vi "GUILib.find control by name.vi"(0 "control name":string, 1 "VIRef":refnum<vi>, 5 "error in (no error)":errorcluster) -> (14 "controlRef":refnum<vi>, 19 "error out":errorcluster)   [LabVIEW 2014, in "GUILib.lvlib"]
doc: "obtains the reference of a control of a VI"
uses:
  GUILib.lvlib
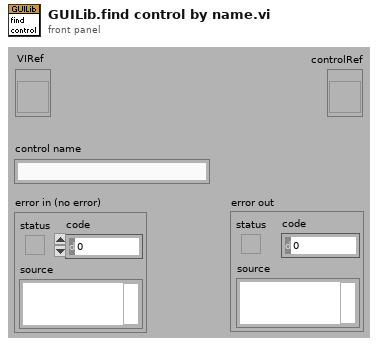
[diagram p1: front panel]
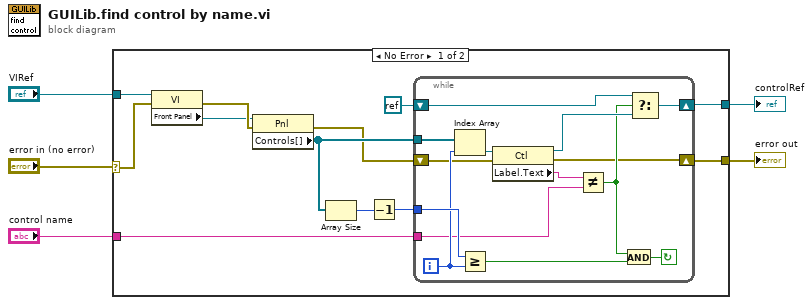
[diagram p0: block diagram]
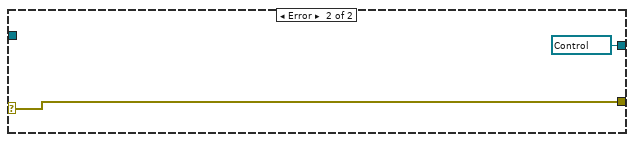
[diagram p2: hidden frame]
diagram:
  n1 = case shown="No Error" "error in (no error)" {
    selector: "error in (no error)" -> [w7 w33]
    tunnel: [w13 refnum<vi> refnum ("dup reference")] -> w5
    tunnel: [w10 w33] -> w4
    tunnel: "VIRef" -> [w9 _]
    tunnel: "control name" -> [w8 _]
    frame No Error {
      n2 = property on="Property Node" class="VI"(reference=w9, error in=w7) -> (error out=w17:errorcluster, "Front Panel"=w16:refnum<vi>)  [unwired: 1 out]
      n3 = property on="Property Node" class="Pnl"(reference=w16, error in=w17) -> (error out=w11:errorcluster, "Controls[]"=w14:refnum<vi>[])  [unwired: 1 out]
      n4 = Array Size(array=w14) -> (size(s)=w15:i32)
      n5 = Decrement(x=w15) -> (x-1=w12:i32)
      n6 = while {
        tunnel: w12 -> [w31]
        tunnel: w14 -> [w30]
        shift-right: [w26] -> w13
        shift-left: refnum<k0> refnum ("Not a Refnum Constant") -> [w25]
        shift-right: [w19] -> w10
        shift-left: w11 -> [w20]
        tunnel: w8 -> [w18]
        i -> [w29]
        stop <- w23 continue-if-true
        n7 = Index Array(array=w30, index=w29) -> (element=w28:refnum<vi>)
        n8 = Greater Or Equal?(x=w31, y=w29) -> (x >= y?=w21:bool)
        n9 = property on="Property Node" class="Ctl"(reference=w28, error in=w20) -> (reference out=w24:refnum<vi>, error out=w19:errorcluster, "Label.Text"=w27:string)
        n10 = Not Equal?(x=w27, y=w18) -> (x != y?=w22:bool)
        n11 = And(x=w22, y=w21) -> (x .and. y?=w23:bool)
        n12 = Select(t=w25, s=w22, f=w24) -> (s? t:f=w26:refnum<vi>)
      }
    }
    frame Error {
    }
  }
  "controlRef" <- w5
  "error out" <- w4
